vi "Vision - Get Current Images.vi"(5 "Printing Report?":bool, 6 "Local Data in":T2 {"Vision Settings"."Dist/Page" items=["Blue (M)/Black (C)", "Red (M)/Green (C)"]}, 7 "UI Refs":T1, 8 "error in (no error)":errorcluster, 11 "Current Distance":dbl) -> (0 "error out":errorcluster, 4 "Local Data out":T2 {"Vision Settings"."Dist/Page" items=["Blue (M)/Black (C)", "Red (M)/Green (C)"]})   [LabVIEW 2024]
uses:
  Controls/Vision - Local Data.ctl
  Controls/Test Cluster.ctl
  Controls/Excluded Information.ctl
  Controls/Language.ctl
  Controls/Device_Type.ctl
  <vilib>/Utility/miscctls.llb/LVRectTypeDef.ctl
  <vilib>/Utility/miscctls.llb/LVBoundsTypeDef.ctl
  Controls/Vision - Reporting Settings.ctl
  Controls/Vision - Dist Per Page.ctl
  Controls/Vision - Section.ctl
  Buttons/Bin.ctl
  Controls/Vision - UI Refs.ctl
  Controls/Vision - Image Dimension Command.ctl
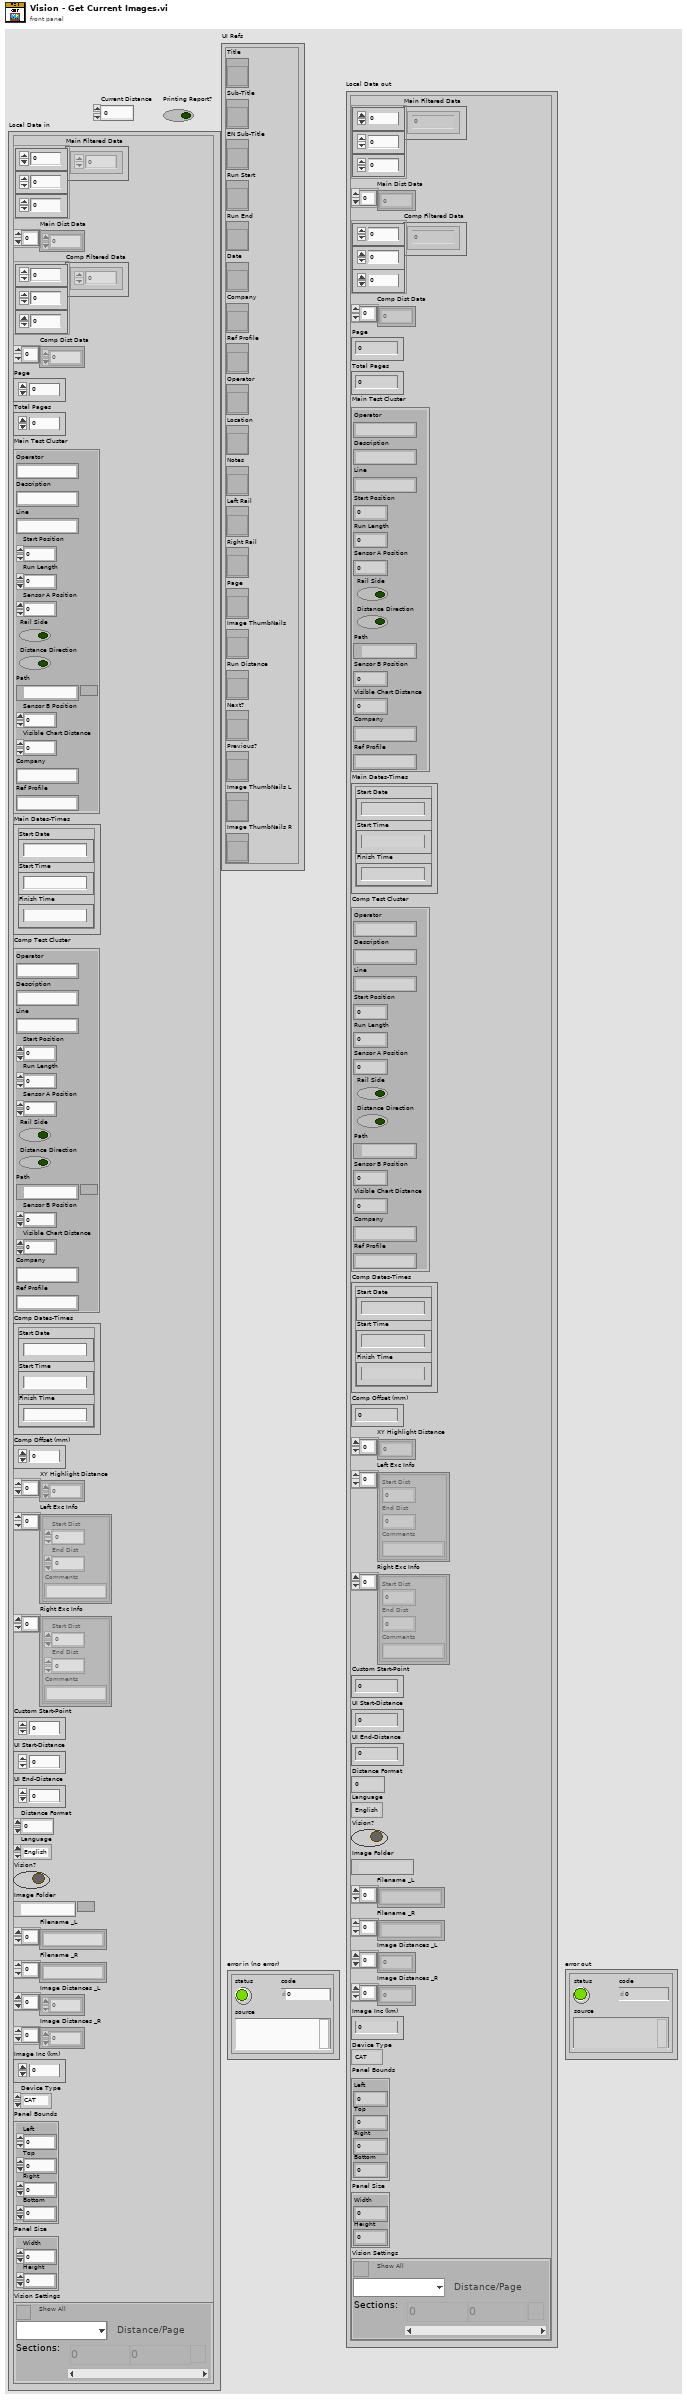
[diagram p1: front panel]
types:
  T1 = typedef "Vision - UI Refs.ctl" = cluster{"Title":refnum<vi>, "Sub-Title":refnum<vi>, "EN Sub-Title":refnum<vi>, "Run Start":refnum<vi>, "Run End":refnum<vi>, "Date":refnum<vi>, "Company":refnum<vi>, "Ref Profile":refnum<vi>, "Operator":refnum<vi>, "Location":refnum<vi>, "Notes":refnum<vi>, "Left Rail":refnum<vi>, "Right Rail":refnum<vi>, "Page":refnum<vi>, "Image ThumbNails":refnum<vi>, "Run Distance":refnum<vi>, "Next?":refnum<vi>, "Previous?":refnum<vi>, "Image ThumbNails L":refnum<vi>, "Image ThumbNails R":refnum<vi>}
  T2 = typedef "Vision - Local Data.ctl" = cluster{"Main Filtered Data":dbl[][][], "Main Dist Data":dbl[], "Comp Filtered Data":dbl[][][], "Comp Dist Data":dbl[], "Page":u8, "Total Pages":u8, "Main Test Cluster":T3, "Main Dates-Times":cluster{"Start Date":string, "Start Time":string, "Finish Time":string}, "Comp Test Cluster":T3, "Comp Dates-Times":cluster{"Start Date":string, "Start Time":string, "Finish Time":string}, "Comp Offset (mm)":i64, "XY Highlight Distance":dbl[], "Left Exc Info":T4[], "Right Exc Info":T4[], "Custom Start-Point":dbl, "UI Start-Distance":dbl, "UI End-Distance":dbl, "Distance Format":u8, "Language":T5, "Vision?":bool, "Image Folder":path, "Filename _L":string[], "Filename _R":string[], "Image Distances _L":dbl[], "Image Distances _R":dbl[], "Image Inc (km)":dbl, "Device Type":T6, "Panel Bounds":T7, "Panel Size":T8, "Vision Settings":T9}
  T3 = typedef "Test Cluster.ctl" = cluster{"Operator":string, "Description":string, "Line":string, "Start Position":dbl, "Run Length":dbl, "Sensor A Position":dbl, "Rail Side":bool, "Distance Direction":bool, "Path":path, "Sensor B Position":dbl, "Visible Chart Distance":dbl, "Company":string, "Ref Profile":string}
  T4 = typedef "Excluded Information.ctl" = cluster{"Start Dist":dbl, "End Dist":dbl, "Comments":string}
  T5 = typedef "Language.ctl" = enum16{"English", "Chinese", "German"}
  T6 = typedef "Device_Type.ctl" = enum16{"CAT", "Bi-CAT", "YRCA", "RCA", "RV-HR", "TV-HR"}
  T7 = typedef "LVRectTypeDef.ctl" = cluster{"Left":i16, "Top":i16, "Right":i16, "Bottom":i16}
  T8 = typedef "LVBoundsTypeDef.ctl" = cluster{"Width":u32, "Height":u32}
  T9 = typedef "Vision - Reporting Settings.ctl" = cluster{"Show All?":bool, "Dist/Page":T10, "Sections":T11[]}
  T10 = typedef "Vision - Dist Per Page.ctl" = u16
  T11 = typedef "Vision - Section.ctl" = cluster{"From":dbl, "To":dbl, "Discard":T12}
  T12 = typedef "Bin.ctl" = bool
  T13 = typedef "Vision - Image Dimension Command.ctl" = enum16{"Get All Dims", "Get # of Images"}
  T14 = typedef "ThumbNail Dimensions.ctl" = cluster{"Row":i32, "Column":i32, "Width Scaling Coeff":dbl, "Height Scaling Coeff":dbl}
  T15 = cluster{"left":i16, "top":i16, "right":i16, "bottom":i16}
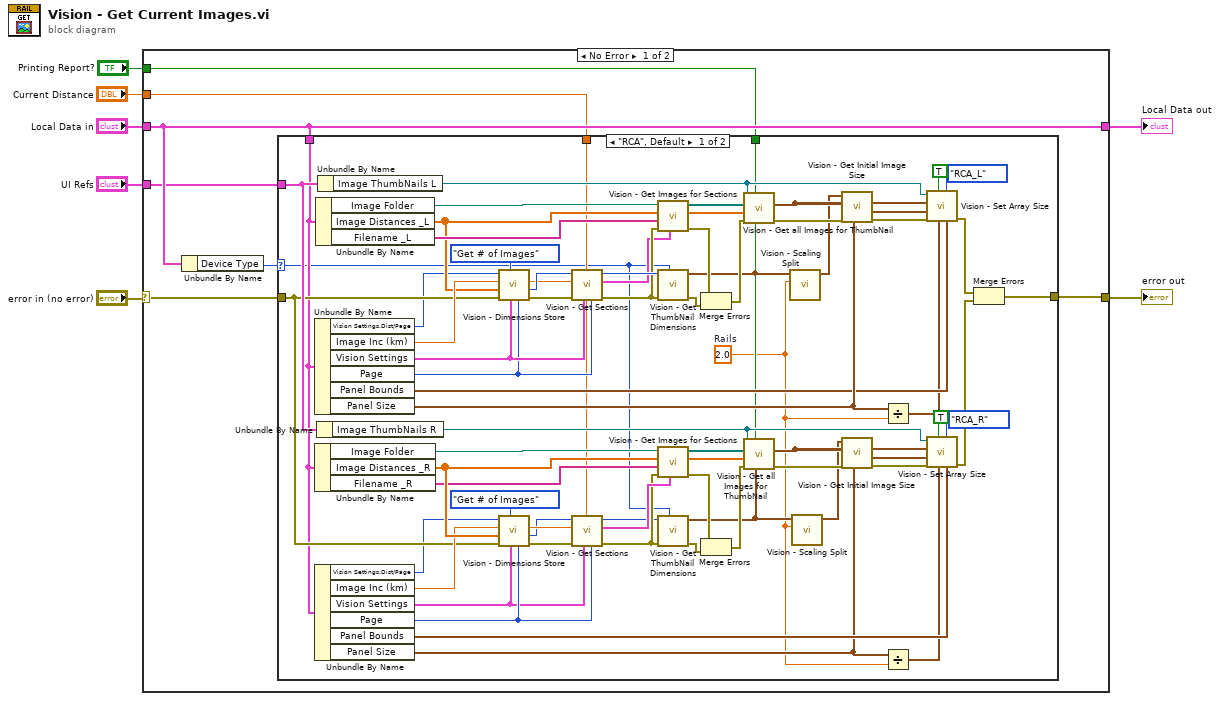
[diagram p0: block diagram]
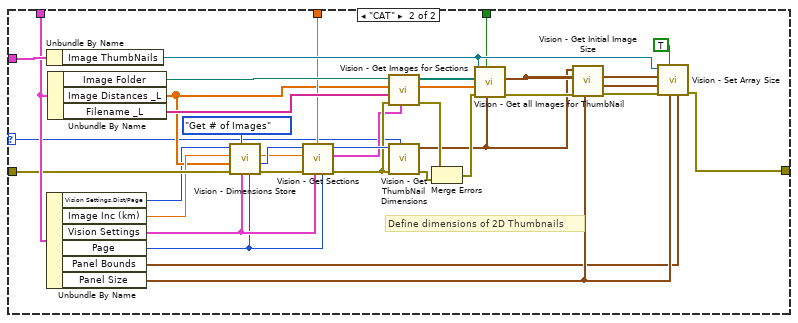
[diagram p2: hidden frame]
diagram:
  n1 = case shown="No Error" "error in (no error)" {
    selector: "error in (no error)" -> [w10 w119]
    tunnel: "UI Refs" -> [w11 _]
    tunnel: [w14 w120] -> w4
    tunnel: "Local Data in" -> [w14 w120]
    tunnel: [w9 w119] -> w7
    tunnel: "Current Distance" -> [w12 _]
    tunnel: "Printing Report?" -> [w8 _]
    frame No Error {
      n2 = Unbundle By Name(w14) -> ("Device Type"=w13:T6)
      n3 = case shown="\"RCA\", Default" w13 {
        selector: w13 -> [w24 w86]
        tunnel: w14 -> [w27 w110]
        tunnel: w12 -> [w31 w98]
        tunnel: w11 -> [w33 w114]
        tunnel: w10 -> [w32 w103]
        tunnel: [w29 w111] -> w9
        tunnel: w8 -> [w30 w88]
        frame "RCA", Default {
          w18 = 2.0  # Rails
          n4 = Unbundle By Name(w27) -> ("Vision Settings.Dist/Page"=w15:T10, "Image Inc (km)"=w68:dbl, "Vision Settings"=w61:T9, "Page"=w60:u8, "Panel Bounds"=w73:T7, "Panel Size"=w74:T8)
          n5 = Unbundle By Name(w27) -> ("Image Folder"=w34:path, "Image Distances _R"=w58:dbl[], "Filename _R"=w35:string[])
          n6 = Unbundle By Name(w27) -> ("Vision Settings.Dist/Page"=w16:T10, "Image Inc (km)"=w49:dbl, "Vision Settings"=w56:T9, "Page"=w57:u8, "Panel Bounds"=w44:T7, "Panel Size"=w43:T8)
          n7 = Unbundle By Name(w27) -> ("Image Folder"=w84:path, "Image Distances _L"=w59:dbl[], "Filename _L"=w83:string[])
          n8 = Unbundle By Name(w33) -> ("Image ThumbNails R"=w42:refnum<vi>)
          n9 = Unbundle By Name(w33) -> ("Image ThumbNails L"=w75:refnum<vi>)
          n10 = call "Vision - Dimensions Store.vi"("Page"=w60, "Supervisory Config Cluster In"=w61, "Command"=Vision_-_Image_Dimension_Command."Get # of Images", "error in (no error)"=w32, "Image Distances _L"=w59, "Inc/page (km)"=w68, "Dist/Page Index"=w15) -> ("error out"=w82:errorcluster, "# of Thumbnails"=w70:i32, "Dist/Page (km)"=w62:dbl)  [unwired: 1 in, 1 out]
          n11 = call "Vision - Dimensions Store.vi"("Page"=w57, "Supervisory Config Cluster In"=w56, "Command"=Vision_-_Image_Dimension_Command."Get # of Images", "error in (no error)"=w32, "Image Distances _L"=w58, "Inc/page (km)"=w49, "Dist/Page Index"=w16) -> ("error out"=w36:errorcluster, "# of Thumbnails"=w47:i32, "Dist/Page (km)"=w55:dbl)  [unwired: 1 in, 1 out]
          n12 = call "Vision - Get Sections.vi"("Page"=w60, "Supervisory Config Cluster In"=w61, "Current Pos (km)"=w31, "error in (no error)"=w82, "Inc/page (km)"=w62) -> ("error out"=w69:errorcluster, "Sections Out"=w67:T11[])  [unwired: 5 in]
          n13 = call "Vision - Get Sections.vi"("Page"=w57, "Supervisory Config Cluster In"=w56, "Current Pos (km)"=w31, "error in (no error)"=w36, "Inc/page (km)"=w55) -> ("error out"=w48:errorcluster, "Sections Out"=w50:T11[])  [unwired: 5 in]
          n14 = call "Vision - Get Images for Sections.vi"("Sections"=w67, "error in (no error)"=w69, "Filename _L"=w83, "Image Distances _L"=w59, "Image Folder in"=w84) -> ("error out"=w63:errorcluster, "Image Distances"=w65:dbl[], "Image Paths"=w66:path[])  [unwired: 4 in]
          n15 = call "Vision - Get ThumbNail Dimensions.vi"("Device Type"=w24, "error in (no error)"=w69, "# of Images"=w70) -> ("error out"=w81:errorcluster, "ThumbNail Dims"=w21:T14)  [unwired: 7 in]
          n16 = call "Vision - Get Images for Sections.vi"("Sections"=w50, "error in (no error)"=w48, "Filename _L"=w35, "Image Distances _L"=w58, "Image Folder in"=w34) -> ("error out"=w54:errorcluster, "Image Distances"=w52:dbl[], "Image Paths"=w51:path[])  [unwired: 4 in]
          n17 = call "Vision - Get ThumbNail Dimensions.vi"("Device Type"=w24, "error in (no error)"=w48, "# of Images"=w47) -> ("error out"=w37:errorcluster, "ThumbNail Dims"=w19:T14)  [unwired: 7 in]
          n18 = Merge Errors(w63, w81) -> (w64:errorcluster)
          n19 = Merge Errors(w54, w37) -> (w53:errorcluster)
          n20 = call "Vision - Get all Images for ThumbNail.vi"("ThumbNail Dims"=w21, "Printing Report?"=w30, "error in (no error)"=w64, "Image Distances"=w65, "ImagePaths"=w66, "Image ThumbNails"=w75) -> ("error out"=w80:errorcluster, "Rectangle"=w76:T15)  [unwired: 4 in]
          n21 = call "Vision - Get all Images for ThumbNail.vi"("ThumbNail Dims"=w19, "Printing Report?"=w30, "error in (no error)"=w53, "Image Distances"=w52, "ImagePaths"=w51, "Image ThumbNails"=w42) -> ("error out"=w38:errorcluster, "Rectangle"=w41:T15)  [unwired: 4 in]
          n22 = call "Vision - Scaling Split.vi"("Rails"=w18, "ThumbNail Dims in"=w21) -> ("ThumbNail Dims out"=w20:T14)  [unwired: 9 in]
          n23 = call "Vision - Scaling Split.vi"("Rails"=w18, "ThumbNail Dims in"=w19) -> ("ThumbNail Dims out"=w17:T14)  [unwired: 9 in]
          n24 = call "Vision - Get Initial Image Size.vi"("Panel Size"=w74, "error in (no error)"=w80, "Rectangle"=w76, "ThumbNail Dims in"=w20) -> ("error out"=w79:errorcluster, "Draw Area Size"=w77:T8)  [unwired: 6 in]
          n25 = call "Vision - Get Initial Image Size.vi"("Panel Size"=w43, "error in (no error)"=w38, "Rectangle"=w41, "ThumbNail Dims in"=w17) -> ("error out"=w39:errorcluster, "Draw Area Size"=w40:T8)  [unwired: 6 in]
          n26 = Divide(x=w74, y=w18) -> (x/y=w26:cluster{"Width":dbl, "Height":dbl})
          n27 = Divide(x=w43, y=w18) -> (x/y=w25:cluster{"Width":dbl, "Height":dbl})
          n28 = call "Vision - Set Array Size.vi"("Panel Bounds"=w73, "Thumbnail?"=enum16{"CAT", "RCA_L", "RCA_R"}."RCA_L", "Panel Size"=w26, "Initialise?"=TRUE, "error in (no error)"=w79, "Draw Area Size"=w77, "Rectangle"=w76, "Image ThumbNails"=w75) -> ("error out"=w78:errorcluster)  [unwired: 3 in]
          n29 = call "Vision - Set Array Size.vi"("Panel Bounds"=w44, "Thumbnail?"=enum16{"CAT", "RCA_L", "RCA_R"}."RCA_R", "Panel Size"=w25, "Initialise?"=TRUE, "error in (no error)"=w39, "Draw Area Size"=w40, "Rectangle"=w41, "Image ThumbNails"=w42) -> ("error out"=w28:errorcluster)  [unwired: 3 in]
          n30 = Merge Errors(w78, w28) -> (w29:errorcluster)
        }
        frame "CAT" {
          # "Define dimensions of 2D Thumbnails"
          n31 = Unbundle By Name(w114) -> ("Image ThumbNails"=w107:refnum<vi>)
          n32 = Unbundle By Name(w110) -> ("Vision Settings.Dist/Page"=w85:T10, "Image Inc (km)"=w99:dbl, "Vision Settings"=w91:T9, "Page"=w90:u8, "Panel Bounds"=w105:T7, "Panel Size"=w106:T8)
          n33 = Unbundle By Name(w110) -> ("Image Folder"=w118:path, "Image Distances _L"=w89:dbl[], "Filename _L"=w117:string[])
          n34 = call "Vision - Dimensions Store.vi"("Page"=w90, "Supervisory Config Cluster In"=w91, "Command"=Vision_-_Image_Dimension_Command."Get # of Images", "error in (no error)"=w103, "Image Distances _L"=w89, "Inc/page (km)"=w99, "Dist/Page Index"=w85) -> ("error out"=w116:errorcluster, "# of Thumbnails"=w101:i32, "Dist/Page (km)"=w92:dbl)  [unwired: 1 in, 1 out]
          n35 = call "Vision - Get Sections.vi"("Page"=w90, "Supervisory Config Cluster In"=w91, "Current Pos (km)"=w98, "error in (no error)"=w116, "Inc/page (km)"=w92) -> ("error out"=w100:errorcluster, "Sections Out"=w97:T11[])  [unwired: 5 in]
          n36 = call "Vision - Get Images for Sections.vi"("Sections"=w97, "error in (no error)"=w100, "Filename _L"=w117, "Image Distances _L"=w89, "Image Folder in"=w118) -> ("error out"=w93:errorcluster, "Image Distances"=w95:dbl[], "Image Paths"=w96:path[])  [unwired: 4 in]
          n37 = call "Vision - Get ThumbNail Dimensions.vi"("Device Type"=w86, "error in (no error)"=w100, "# of Images"=w101) -> ("error out"=w115:errorcluster, "ThumbNail Dims"=w87:T14)  [unwired: 7 in]
          n38 = Merge Errors(w93, w115) -> (w94:errorcluster)
          n39 = call "Vision - Get all Images for ThumbNail.vi"("ThumbNail Dims"=w87, "Printing Report?"=w88, "error in (no error)"=w94, "Image Distances"=w95, "ImagePaths"=w96, "Image ThumbNails"=w107) -> ("error out"=w113:errorcluster, "Rectangle"=w108:T15)  [unwired: 4 in]
          n40 = call "Vision - Get Initial Image Size.vi"("Panel Size"=w106, "error in (no error)"=w113, "Rectangle"=w108, "ThumbNail Dims in"=w87) -> ("error out"=w112:errorcluster, "Draw Area Size"=w109:T8)  [unwired: 6 in]
          n41 = call "Vision - Set Array Size.vi"("Panel Bounds"=w105, "Panel Size"=w106, "Initialise?"=TRUE, "error in (no error)"=w112, "Draw Area Size"=w109, "Rectangle"=w108, "Image ThumbNails"=w107) -> ("error out"=w111:errorcluster)  [unwired: 4 in]
        }
      }
    }
    frame Error {
    }
  }
  "error out" <- w7
  "Local Data out" <- w4
